vi "Close.vi"(8 "Error In":errorcluster, 11 "LINX Resource":T1) -> (0 "Error Out":errorcluster)   [LabVIEW 2020, in "LMH-LINX.lvlib"]
doc: "Close the connection to the remote LINX device and free any local I/O resources."
uses:
  LMH-LINX.lvlib
  Private/Type Defs/LINX Ref.ctl
  Private/Type Defs/Platform.ctl
  Private/Type Defs/Interface.ctl
  Private/Device/Type Defs/LINX Device Config.ctl
  Private/Device/Type Defs/TCP Config.ctl
  Private/Device/Type Defs/Channels.ctl
  Private/Device/Device.lvlib
  Private/Local IO/Local IO.lvlib
panel:
  out "Error Out 2":errorcluster
  out "LINX Resource":T1
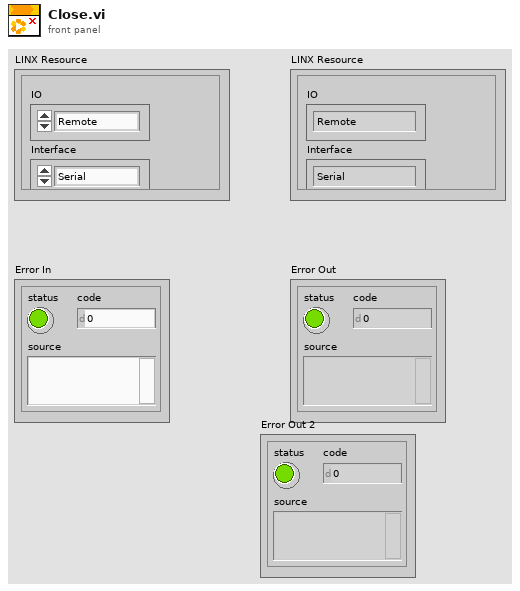
[diagram p1: front panel]
types:
  T1 = typedef "LMH-LINX.lvlib/LINX Ref.ctl" = cluster{"IO":T2, "Interface":T3, "LINX Device Config":T4}
  T2 = typedef "LMH-LINX.lvlib/Platform.ctl" = enum16{"Remote", "Local"}
  T3 = typedef "LMH-LINX.lvlib/Interface.ctl" = enum16{"Serial", "TCP"}
  T4 = typedef "LMH-LINX.lvlib/Device.lvlib/LINX Device Config.ctl" = cluster{"Interface":T3, "COM Port":refnum<visa-resource-name>, "TCP Configuration":T5, "Device Family":u8, "Device ID":u8, "Device Name":string, "TCP Ref":refnum<k5>, "Channels":T6}
  T5 = typedef "LMH-LINX.lvlib/Device.lvlib/TCP Config.ctl" = cluster{"IP Address":string, "Port":u16}
  T6 = typedef "LMH-LINX.lvlib/Channels.ctl" = cluster{"DI":u8[], "DO":u8[], "AI":u8[], "AO":u8[], "PWM":u8[], "QE":u8[], "UART":u8[], "I2C 2":u8[], "SPI":u8[], "CAN":u8[], "Servo":u8[], "AI Ref (V)":dbl, "AI Resolution (Bits)":u8, "AO Ref (V)":dbl, "AO Resolution (Bits)":u8}
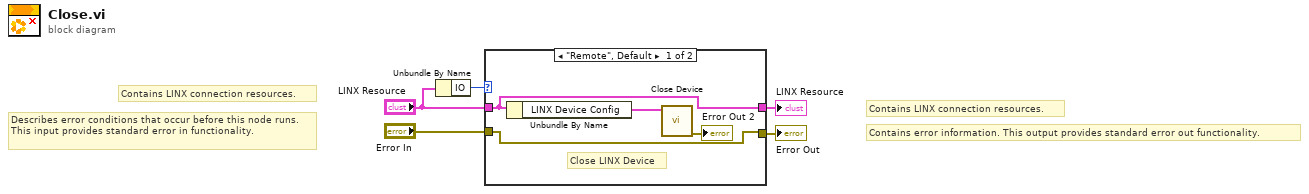
[diagram p0: block diagram]
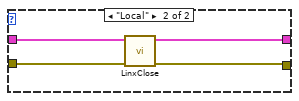
[diagram p2: hidden frame]
diagram:
  # "Contains LINX connection resources."
  # "Describes error conditions that occur before this node runs. This input provides standard error in functionality."
  # "Contains error information. This output provides standard error out functionality."
  # "Contains LINX connection resources."
  n1 = Unbundle By Name("LINX Resource") -> ("IO"=w5:T2)
  n2 = case shown="\"Remote\", Default" w5 {
    tunnel: "LINX Resource" -> [w8 w10]
    tunnel: [w8 w11] -> w3
    tunnel: [w7 w12] -> w2
    tunnel: "Error In" -> [w7 w13]
    frame "Remote", Default {
      # "Close LINX Device"
      n3 = Unbundle By Name(w8) -> ("LINX Device Config"=w9:T4)
      n4 = call "Close Device.vi"("LINX Device Config"=w9) -> ("Error Out"=→"Error Out 2":errorcluster)  [unwired: 9 in, 1 out]
    }
    frame "Local" {
      n5 = call "LinxClose.vi"("Error In"=w13, "LINX Resource"=w10) -> ("Error Out"=w12:errorcluster, "LINX Resource"=w11:T1)  [unwired: 8 in]
    }
  }
  "Error Out" <- w2
  "LINX Resource" <- w3
